vi "Calc_clean.vi"(8 "error in (no error)":errorcluster, 10 "Clean mode":enum32{"delete", "approx"}(ring), 11 "Control-Client in":refnum<class "Control-Client.lvclass">) -> (0 "error out":errorcluster, 1 "Experiment.lvclass out":refnum<class "Experiment.lvclass">, 2 "Data out":dbl[][](array[numeric]), 3 "Control-Client out":refnum<class "Control-Client.lvclass">, 5 "timedelays old":dbl[](array[numeric]))   [LabVIEW 2020, in "Control-Client.lvclass"]
uses:
  Control-Client.lvclass
  Experiments/Experiment.lvclass
  Control-Client.lvclass/Control-Client.ctl
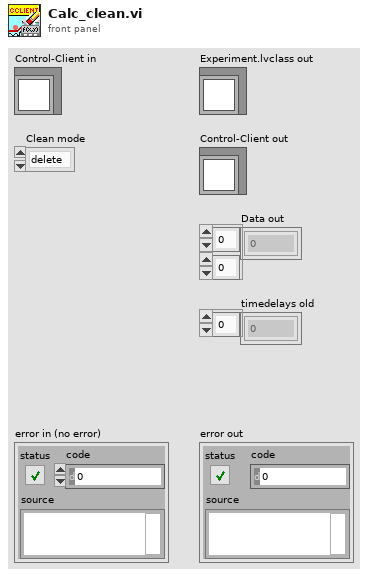
[diagram p1: front panel]
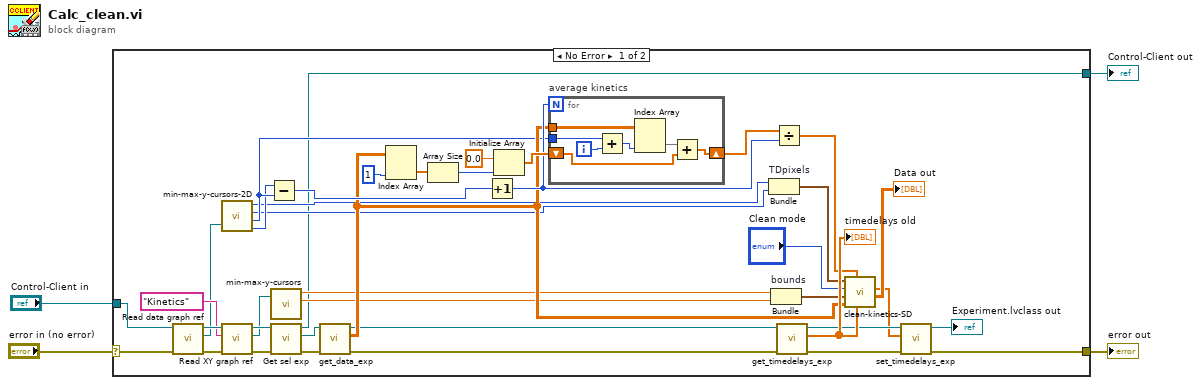
[diagram p0: block diagram]
diagram:
  n1 = case shown="No Error" "error in (no error)" {
    selector: "error in (no error)" -> [w6 w52]
    tunnel: "Control-Client in" -> [w38 w53]
    tunnel: [w8 w52] -> w3
    tunnel: [w7 w53] -> w2
    frame No Error {
      n2 = call "Read data graph ref.vi"("error in (no error)"=w6, "Control-Client in"=w38) -> ("error out"=w42:errorcluster, "Exp data graph ref"=w32:refnum<vi>, "Control-Client out"=w40:refnum<class "Control-Client.lvclass">)  [unwired: 7 in]
      n3 = call "min-max-y-cursors-2D.vi"("GRAPH EXPERIMENTAL DATA ref"=w32) -> ("minY"=w15:i32, "maxY"=w14:i32, "minX"=w21:i32, "maxX"=w20:i32)  [unwired: 1 in]
      n4 = call "Read XY graph ref.vi"("error in (no error)"=w42, "Combo Box"="Kinetics", "Control-Client in"=w40) -> ("error out"=w43:errorcluster, "XY graph ref"=w33:refnum<vi>, "Control-Client out"=w41:refnum<class "Control-Client.lvclass">)  [unwired: 6 in]
      n5 = Subtract(x=w20, y=w21) -> (x-y=w25:i32)
      n6 = call "min-max-y-cursors.vi"("XYGraph in"=w33) -> ("minY"=w17:dbl, "maxY"=w16:dbl)  [unwired: 1 in, 2 out]
      n7 = call "Get sel exp.vi"("error in (no error)"=w43, "Control-Client in"=w41) -> ("error out"=w44:errorcluster, "Sel experiment"=w37:refnum<class "Experiment.lvclass">, "Control-Client out"=w7:refnum<class "Control-Client.lvclass">)  [unwired: 7 in]
      n8 = call "get_data_exp.vi"("error in (no error)"=w44, "Experiment.lvclass in"=w37) -> ("error out"=w18:errorcluster, "Data"=w23:sgl[][], "Experiment.lvclass out"=w19:refnum<class "Experiment.lvclass">)  [unwired: 7 in]
      n9 = Index Array(array=w23, index (col)=1 ("disabled index (col)")) -> (element=w27:sgl[])  [unwired: 1 in]
      n10 = Array Size(array=w27) -> (size(s)=w29:i32)
      n11 = Increment(x=w25) -> (x+1=w24:i32)
      n12 = Initialize Array(0.0 ("element"), w29) -> (w26:dbl[])
      n13 = for "average kinetics" {
        N: w24 -> [_]
        tunnel: w23 -> [w51]
        shift-right: [w46] -> w30
        shift-left: w26 -> [w47]
        tunnel: w21 -> [w45]
        i -> [w50]
        n14 = Add(x=w45, y=w50) -> (x+y=w49:i32)
        n15 = Index Array(array=w51, index (col)=w49) -> (element=w48:sgl[])  [unwired: 1 in]
        n16 = Add(x=w48, y=w47) -> (x+y=w46:dbl[])
      }
      n17 = Bundle "TDpixels"("minY"=w15, "maxY"=w14) -> (w12:cluster{"minY":i32, "maxY":i32})  [unwired: 1 in]
      n18 = Bundle "bounds"("minY"=w17, "maxY"=w16) -> (w13:cluster{"minY":dbl, "maxY":dbl})  [unwired: 1 in]
      n19 = Divide(x=w30, y=w24) -> (x/y=w22:dbl[])
      n20 = call "get_timedelays_exp.vi"("error in (no error)"=w18, "Experiment.lvclass in"=w19) -> ("error out"=w10:errorcluster, "timedelays"=w39:dbl[], "Experiment.lvclass out"=w11:refnum<class "Experiment.lvclass">)  [unwired: 7 in]
      "timedelays old" <- w39
      n21 = call "clean-kinetics-SD.vi"("timedelays"=w39, "kinetics"=w22, "Data"=w23, "bounds"=w13, "Clean mode"="Clean mode", "TDpixels"=w12) -> ("Data out"=→"Data out":dbl[][], "timedelays out"=w5:dbl[])  [unwired: 3 in]
      n22 = call "set_timedelays_exp.vi"("error in (no error)"=w10, "timedelays"=w5, "Experiment.lvclass in"=w11) -> ("error out"=w8:errorcluster, "Experiment.lvclass out"=→"Experiment.lvclass out":refnum<class "Experiment.lvclass">)  [unwired: 7 in]
    }
    frame Error {
    }
  }
  "error out" <- w3
  "Control-Client out" <- w2
